vi "_CSM Message Communication Panel.vi"() -> ()   [LabVIEW 2017]
uses:
  user.lib/_NEVSTOP/Communicable State Machine(CSM)/_Support/Typedef/_CSM_GlobalLog_MSG.ctl
  user.lib/_NEVSTOP/Communicable State Machine(CSM)/_Support/Typedef/_CSM_Response Source Message.ctl
  user.lib/_NEVSTOP/Communicable State Machine(CSM)/_Support/Typedef/_CSM_GlobalLog_MSG_TYPE.ctl
  user.lib/_NEVSTOP/Communicable State Machine(CSM)/_Polymophic/Add State(s) to Queue By BOOL(Element).vi
  230fd0d1-fada-4a8e-b720-9cb1801ca748.vi
  70dded23-6362-40d9-8646-ef12445fa2f7.vi
  user.lib/_NEVSTOP/Communicable State Machine(CSM)/_Polymophic/Build Synchronous Message with Arguments.vi
  user.lib/_NEVSTOP/Communicable State Machine(CSM)/_Polymophic/Build No-Reply Asynchronous Message with Arguments.vi
  user.lib/_NEVSTOP/Communicable State Machine(CSM)/AdvanceAPI/CSM - Keywords.vi
  user.lib/_NEVSTOP/Communicable State Machine(CSM)/AdvanceAPI/CSM - Convert Error to Argument.vi
  user.lib/_NEVSTOP/Communicable State Machine(CSM)/_Support/GlobalEvent/GEvt-Generate with Rule Check.vi
  user.lib/_NEVSTOP/Communicable State Machine(CSM)/_Support/Message/Parse State with Arguments String.vi
  <vilib>/Utility/config.llb/Close Config Data.vi
  <vilib>/Utility/config.llb/Write Key.vi
  <vilib>/Utility/config.llb/Write Key (Double).vi
  <vilib>/Utility/config.llb/Write Key (I32).vi
  <vilib>/Utility/config.llb/Write Key (String).vi
  user.lib/_NEVSTOP/Communicable State Machine(CSM)/_csmHelper/lvcsmFile/Path to lvcsm String.vi
  <vilib>/Utility/config.llb/Remove Key.vi
  <vilib>/Utility/config.llb/Get Key Names.vi
  <vilib>/Utility/Data Type/Get Type Information.vi
  <vilib>/Utility/Data Type/Get Array Information.vi
  <vilib>/Utility/config.llb/Write Key (Boolean).vi
  <vilib>/Utility/config.llb/Open Config Data.vi
  user.lib/_NEVSTOP/Communicable State Machine(CSM)/_csmHelper/lvcsmFile/lvcsm File Path.vi
  user.lib/_NEVSTOP/Communicable State Machine(CSM)/_csmHelper/lvcsmFile/_Array of VData to VCluster.vi
  <vilib>/Utility/config.llb/Read Key.vi
  <vilib>/Utility/config.llb/Read Key (Double).vi
  <vilib>/Utility/config.llb/Read Key (I32).vi
  user.lib/_NEVSTOP/Communicable State Machine(CSM)/_csmHelper/lvcsmFile/lvcsm String to Path.vi
  <vilib>/Utility/config.llb/Read Key (String).vi
  <vilib>/Utility/config.llb/Read Key (Boolean).vi
  user.lib/_NEVSTOP/Communicable State Machine(CSM)/_Support/GlobalEvent/LogFilter/LogFilter - Check.vi
  user.lib/_NEVSTOP/Communicable State Machine(CSM)/_Support/GlobalEvent/Cache-GEvt Refs.vi
  user.lib/_NEVSTOP/Communicable State Machine(CSM)/_Support/GlobalEvent/LogFilter/LogFilter.lvclass
  user.lib/_NEVSTOP/Communicable State Machine(CSM)/Communicable State Machine.lvlib
  user.lib/_NEVSTOP/Communicable State Machine(CSM)/_Shared/CSM Shared.lvlib
panel:
  in  "History":i32(listbox)
  in  "CSM 2":string(combo)
  in  "Refresh":bool
  in  "Arguments":string
  out "Response":string
  in  "Clear History":bool
  in  "History Length":i32=50 min=20 max=1000 step=1
  in  "CSM":string(combo)
  in  "Refresh CSM":bool
  in  "RespTMO(ms)":i32=10000 format="%.0p"
  in  "Sync (-@) 2":bool
  in  "Sync (-@)":bool
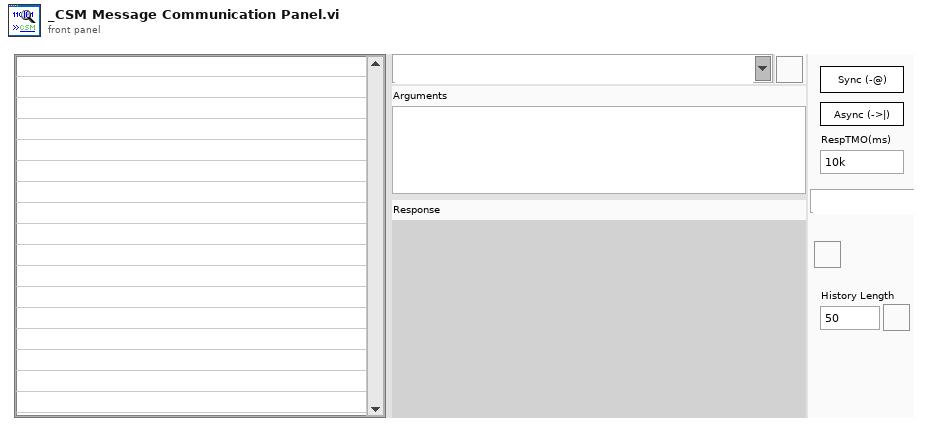
[diagram p1: front panel]
types:
  T1 = enum32{"Invalid", "Standard", "Closed", "Hidden", "Minimized", "Maximized"}
  T2 = enum32{"invalid app kind", "Development System", "Run Time System", "Student Edition", "Embedded LabVIEW", "Evaluation", "Custom"}
  T3 = cluster{"Response Timeout(ms)":i32, "History Length":i32, "History":string[]}
  T4 = cluster{"Shift":bool, "Ctrl":bool, "Alt":bool, "Cmd":bool, "Opt":bool}
  T5 = cluster{"Core":cluster{"Current VI Reference":refnum<vi>, "Close Panel on Exit?":bool}, "CSM Global Log Event":refnum<user-event>, "MessageList":string[], "Toobar.advance":refnum<vi>[]}
  T6 = typedef "LVPoint32TypeDef.ctl" = cluster{"Horizontal":i32, "Vertical":i32}
  T7 = cluster{"Current VI Reference":refnum<vi>, "Close Panel on Exit?":bool}
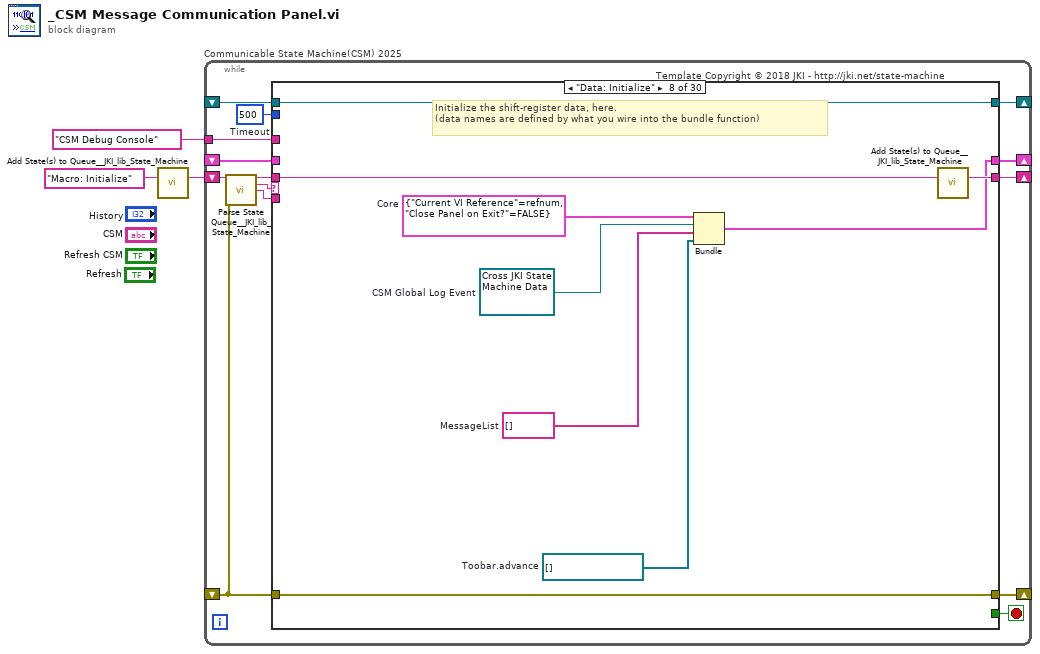
[diagram p0: block diagram]
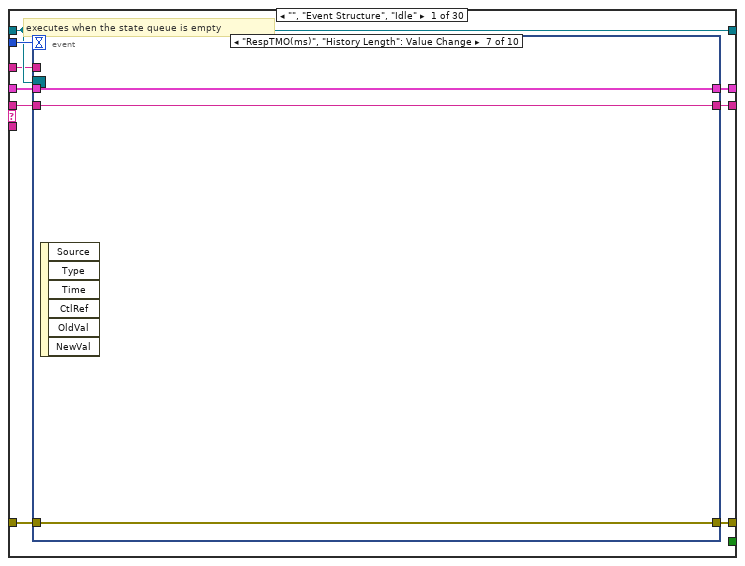
[diagram p2: hidden frame]
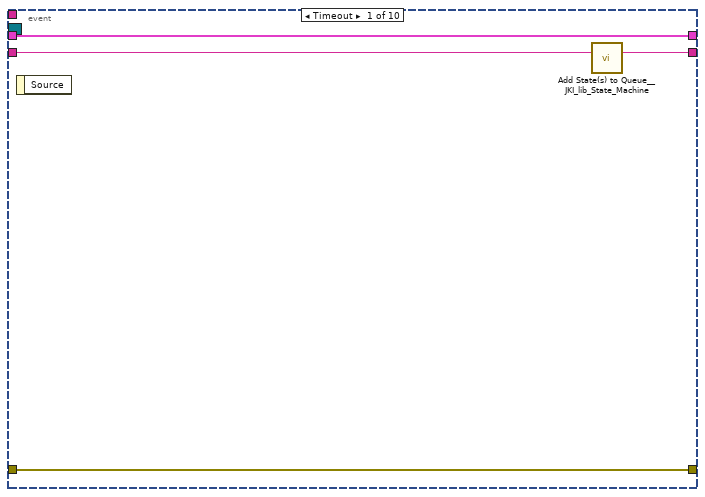
[diagram p3: hidden frame]
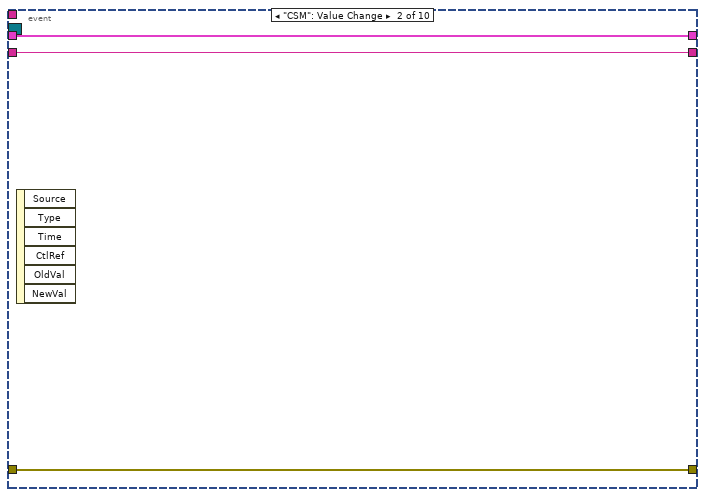
[diagram p4: hidden frame]
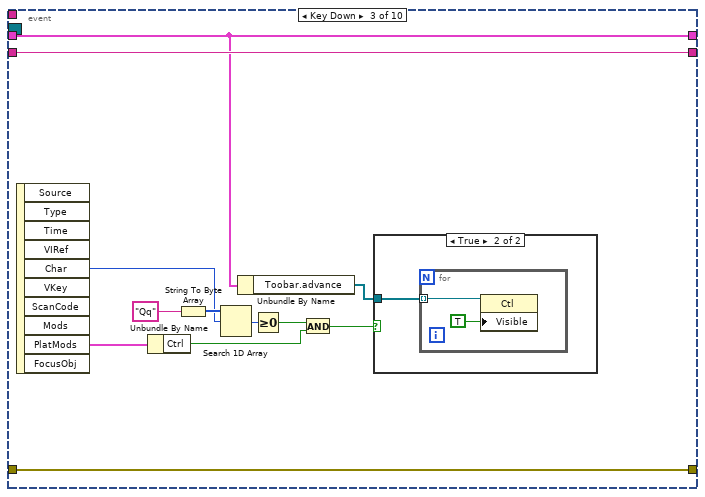
[diagram p5: hidden frame]
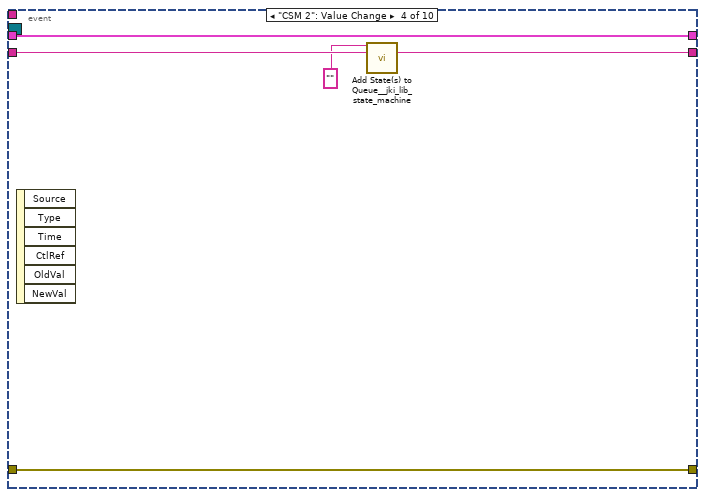
[diagram p7: hidden frame]
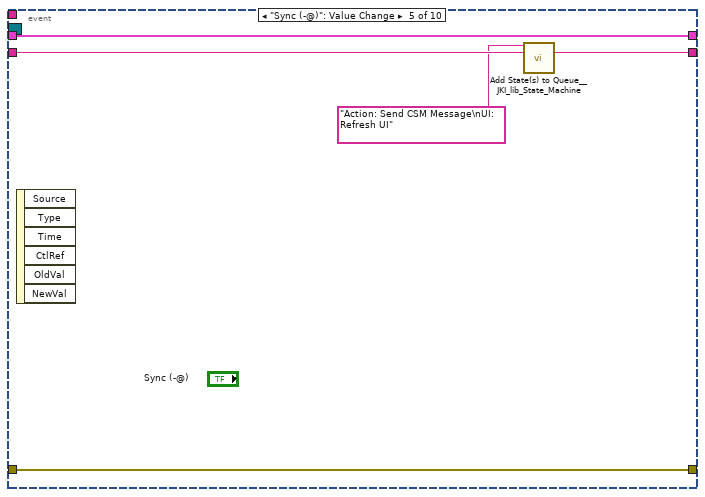
[diagram p8: hidden frame]
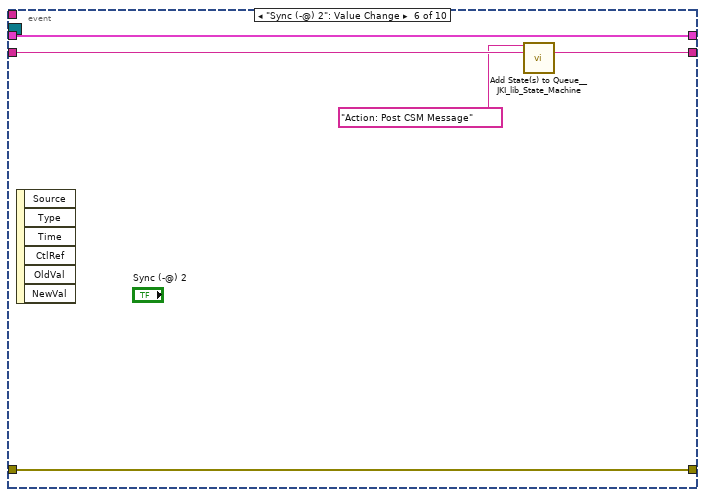
[diagram p9: hidden frame]
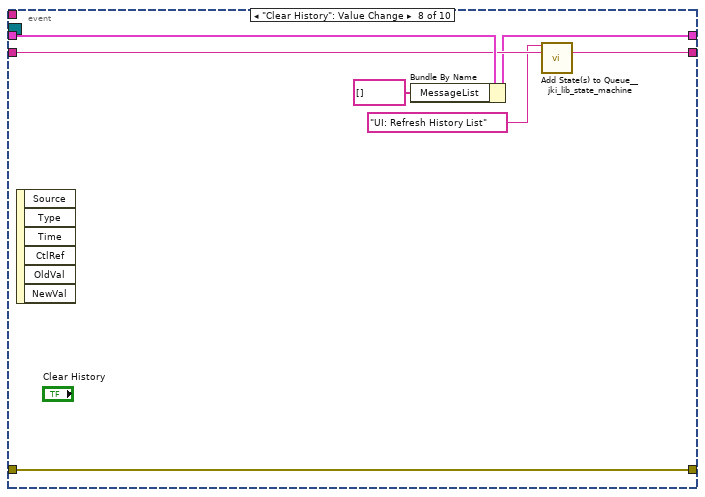
[diagram p10: hidden frame]
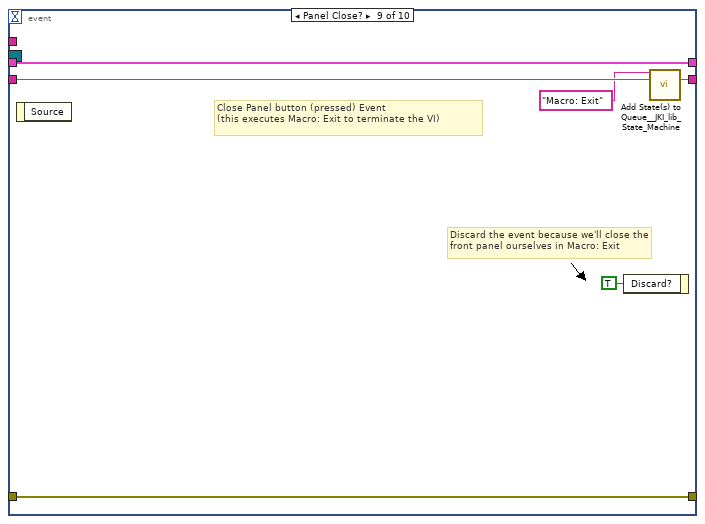
[diagram p11: hidden frame]
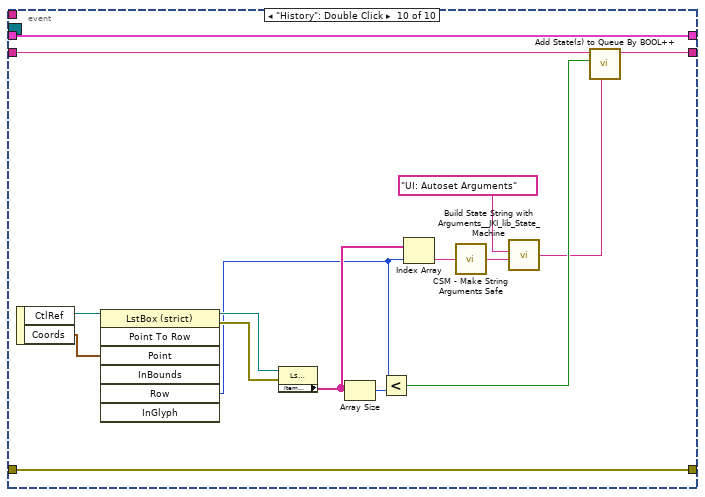
[diagram p12: hidden frame]
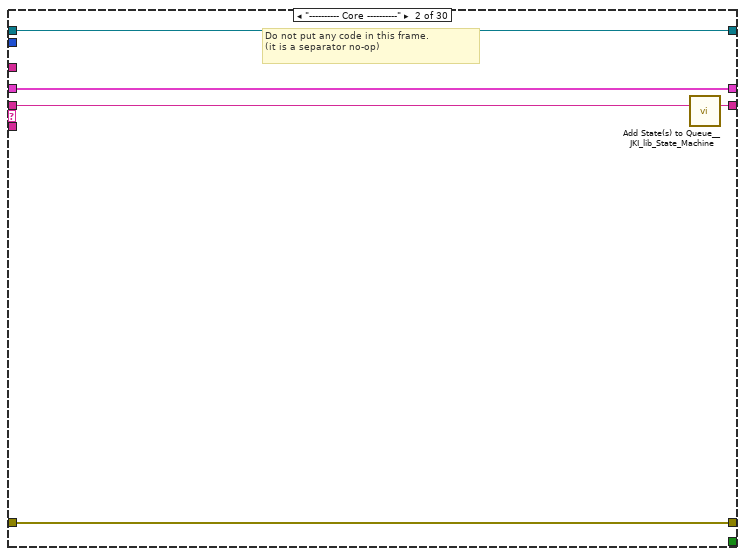
[diagram p13: hidden frame]
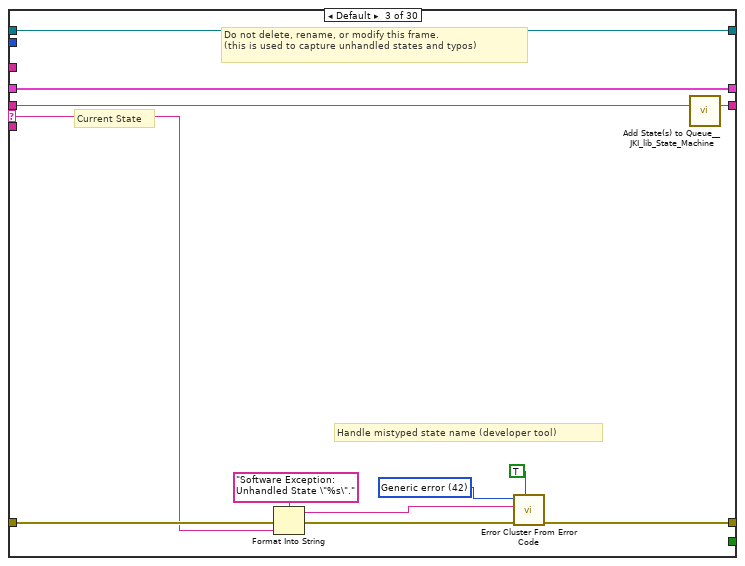
[diagram p14: hidden frame]
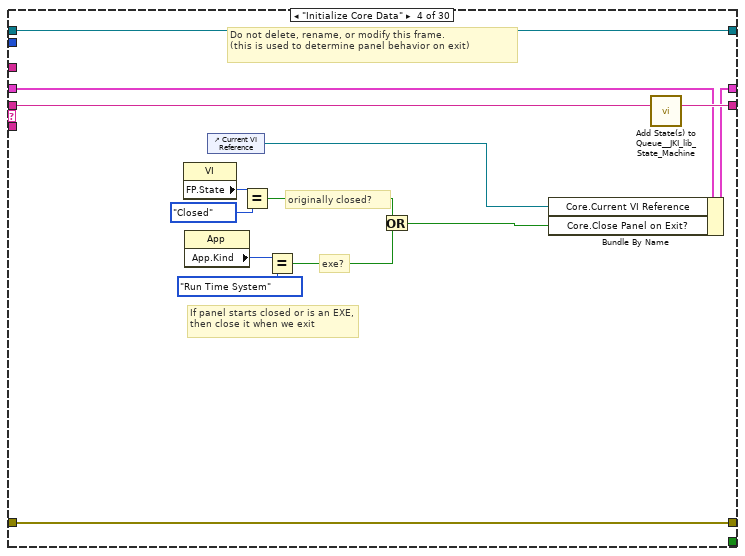
[diagram p15: hidden frame]
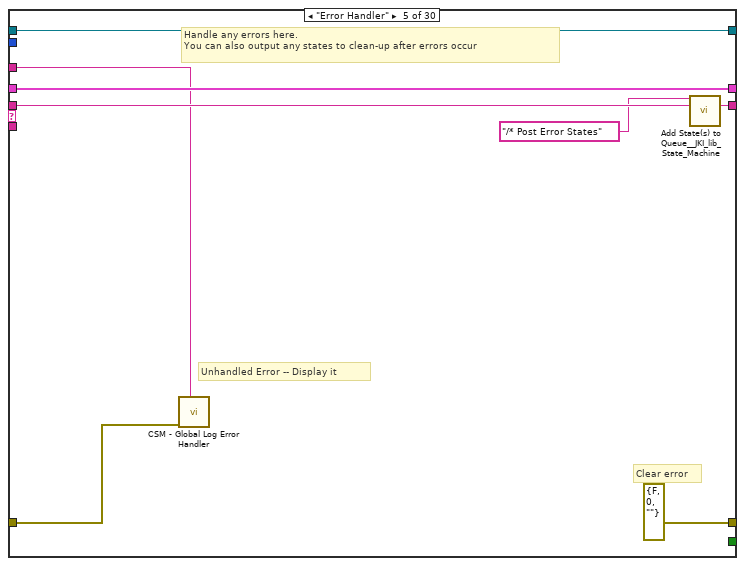
[diagram p16: hidden frame]
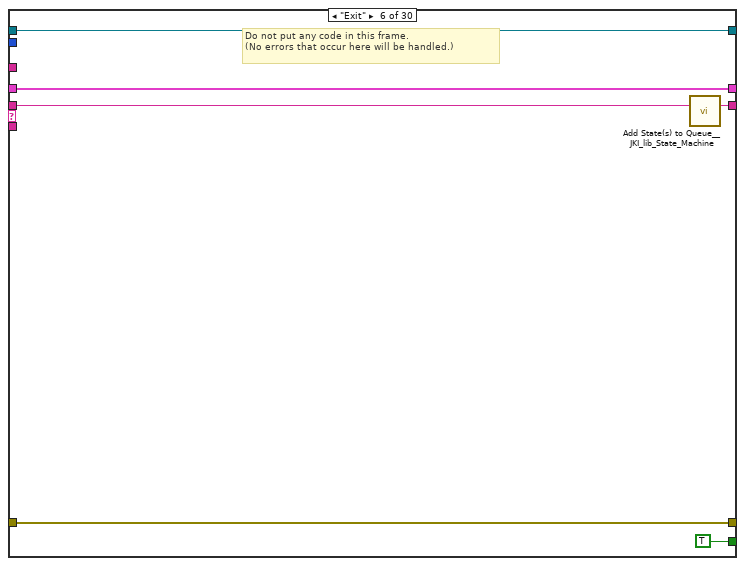
[diagram p17: hidden frame]
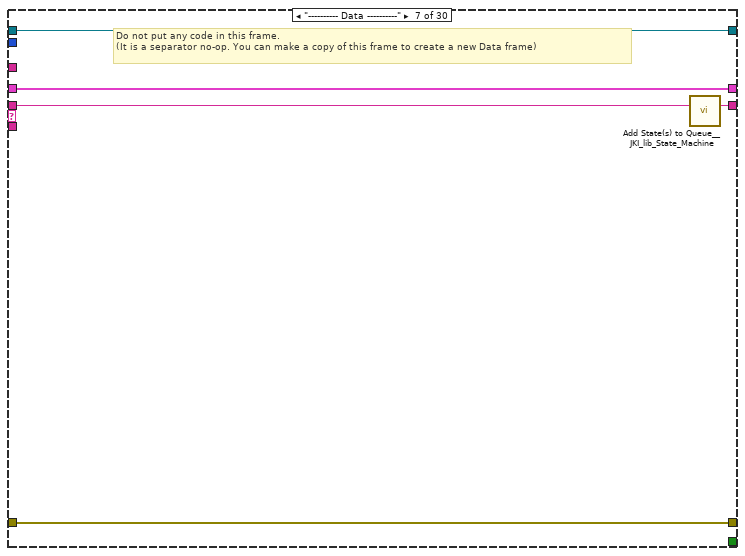
[diagram p18: hidden frame]
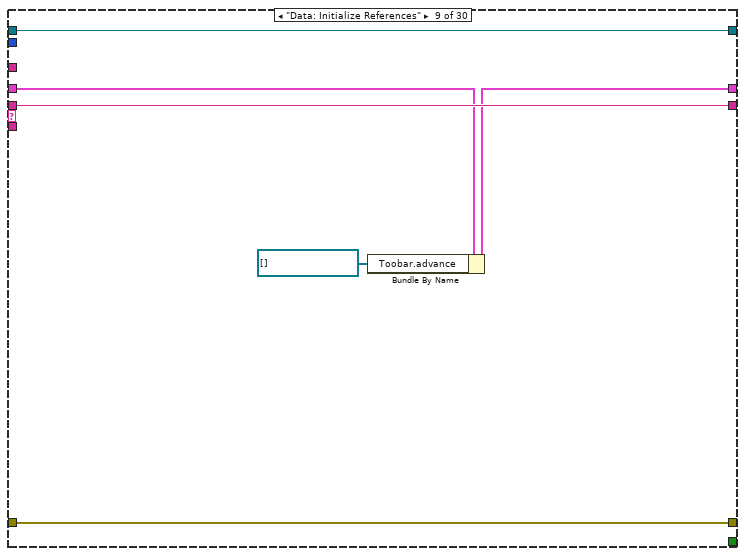
[diagram p19: hidden frame]
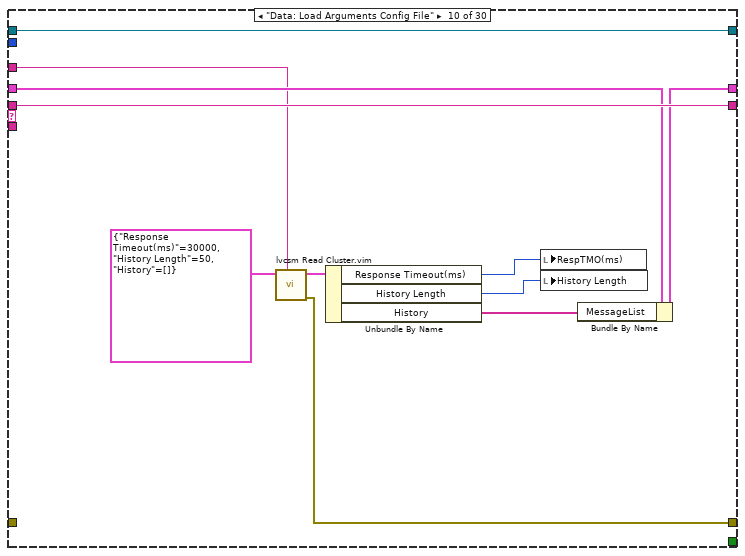
[diagram p20: hidden frame]
diagram:
  n1 = call <vilib>:"Add State(s) to Queue__JKI_lib_State_Machine.vi"("State(s) in (\"\")"="Macro: Initialize") -> ("States Out"=w2:string)  [unwired: 14 in]
  n2 = while "Communicable State Machine(CSM) 2025" {
    shift-right: [w10] -> _
    shift-left: _ -> [w9]
    shift-right: [w13] -> _
    shift-left: _ -> [w7]
    shift-right: [w12] -> _
    shift-left: w2 -> [w14]
    shift-right: [w6] -> _
    shift-left: _ -> [w5]
    tunnel: "CSM Debug Console" -> [w4]
    stop <- w11 stop-if-true
    w8 = 500  # Timeout
    # "Template Copyright © 2018 JKI - http://jki.net/state-machine"
    n3 = call <vilib>:"Parse State Queue__JKI_lib_State_Machine.vi"("State Queue"=w14, "Error In (no error)"=w7) -> ("Remaining States"=w16:string, "Current State"=w17:string, "Arguments"=w15:string)  [unwired: 11 in]
    n4 = case shown="\"Data: Initialize\"" w17 {
      selector: w17 -> [_ _ w102 _ _ _ _ _ _ _ _ _ _ _ _ _ _ _ _ _ _ _ _ _ _ _ _ _ _ _]
      tunnel: w16 -> [w26 w100 w106 w126 w134 w140 w145 w154 w159 w171 w181 w194 w210 w215 w222 w229 w234 w240 w250 w262 w341 w352 w365 w369 w375 w381 w392 w397 w407 w429]
      tunnel: w15 -> [_ _ _ _ _ _ _ _ _ _ _ w189 _ _ _ _ _ _ w245 w256 w339 _ _ _ _ _ _ _ _ _]
      tunnel: w9 -> [w24 w97 w104 w119 w131 w138 w142 _ w158 w168 w179 w191 w205 w212 w220 w225 w231 w236 w248 w258 w336 w350 w364 w367 w372 w378 w389 w394 w405 w427]
      tunnel: [w23 w98 w108 w123 errorcluster {"status"=FALSE, "code"=0, "source"=""} ("error out") w137 w143 w151 w160 w164 w174 w192 w206 w213 w218 w226 w232 w238 w246 w259 w342 w353 w366 w370 w373 w379 w390 w395 w401 w425] -> w13
      tunnel: w7 -> [w22 w98 w107 w123 w130 w137 w143 w151 w160 _ _ w192 w207 w213 _ _ w232 w238 w247 w260 w342 w353 w366 w370 w373 w379 w390 w395 _ _]
      tunnel: [w25 w99 w105 w125 w133 w139 w144 w153 w159 w171 w181 w194 w209 w214 w221 w228 w233 w239 w249 w261 w341 w352 w365 w369 w374 w380 w391 w396 w406 w428] -> w12
      tunnel: [_ _ _ _ _ TRUE _ _ _ _ _ _ _ _ _ _ _ _ _ _ _ _ _ _ _ _ _ _ _ _] -> w11
      tunnel: [w21 w97 w104 w124 w131 w138 w142 w152 w156 w169 w179 w185 w205 w212 w220 w225 w231 w236 w248 w258 w336 w350 w364 w367 w372 w378 w389 w394 w405 w427] -> w10
      tunnel: w8 -> [w20 _ _ _ _ _ _ _ _ _ _ _ _ _ _ _ _ _ _ _ _ _ _ _ _ _ _ _ _ _]
      tunnel: [w19 w96 w101 w113 w128 w135 w141 w149 w157 w170 w180 w193 w204 w211 w219 w227 w230 w237 w244 w255 w340 w351 w363 w368 w371 w376 w382 w393 w404 w426] -> w6
      tunnel: w5 -> [w19 w96 w101 w113 w128 w135 w141 w149 w157 w170 w180 w193 w204 w211 _ w227 w230 w237 w244 w255 w340 w351 w363 w368 w371 w376 w382 w393 w404 w426]
      tunnel: w4 -> [w18 _ _ _ w127 _ _ _ _ w163 w175 _ _ _ _ _ _ _ _ _ _ _ _ _ _ _ _ _ _ _]
      frame "", "Event Structure", "Idle" {
        # "executes when the state queue is empty"
        n5 = event shown="[6] \"RespTMO(ms)\", \"History Length\": Value Change" {
          selector: w19 -> [_ _ _ _ _ _ _ _ _ _]
          dyn-events: _ -> [_ _ _ _ _ _ _ _ _ _]
          timeout: w20 -> [_ _ _ _ _ _ _ _ _ _]
          tunnel: w26 -> [w30 w33 w45 w50 w55 w60 w66 w70 w79 w87]
          tunnel: [w29 w33 w45 w51 w56 w61 w66 w71 w78 w88] -> w25
          tunnel: w24 -> [w27 w31 w34 w52 w57 w62 w64 w72 w76 w94]
          tunnel: [w28 w32 w44 w53 w58 w63 w65 w73 w77 w95] -> w23
          tunnel: w22 -> [w28 w32 w44 w53 w58 w63 w65 w73 w77 w95]
          tunnel: [w27 w31 w34 w52 w57 w62 w64 w68 w76 w94] -> w21
          tunnel: w18 -> [_ _ _ _ _ _ _ _ _ _]
          event Timeout {
            n6 = event-data() -> ()  [unwired: 1 in, 1 out]
            n7 = call <vilib>:"Add State(s) to Queue__JKI_lib_State_Machine.vi"("State(s) in (\"\")"=w30) -> ("States Out"=w29:string)  [unwired: 14 in]
          }
          event "CSM": Value Change {
            n8 = event-data() -> ()  [unwired: 1 in, 6 out]
          }
          event Key Down {
            n9 = event-data() -> ("Char"=w35:i16, "PlatMods"=w36:T4)  [unwired: 1 in, 8 out]
            n10 = Unbundle By Name(w36) -> ("Ctrl"=w39:bool)
            n11 = String To Byte Array(string="Qq") -> (unsigned byte array=w41:u8[])
            n12 = Search 1D Array(1D array=w41, element=w35) -> (index of element=w42:i32)  [unwired: 1 in]
            n13 = Unbundle By Name(w34) -> ("Toobar.advance"=w37:refnum<vi>[])
            n14 = Greater Or Equal To 0?(x=w42) -> (x >= 0?=w43:bool)
            n15 = And(x=w43, y=w39) -> (x .and. y?=w38:bool)
            n16 = case shown="True" w38 {
              tunnel: w37 -> [_ w46]
              frame False {
              }
              frame True {
                n17 = for {
                  tunnel: w46 -> [w48] mode=indexing
                  n18 = property class="Ctl"(reference=w48, "Visible"=TRUE) -> ()  [unwired: 1 in, 2 out]
                }
              }
            }
          }
          event "CSM 2": Value Change {
            n19 = event-data() -> ()  [unwired: 1 in, 6 out]
            n20 = call <vilib>:"Add State(s) to Queue__jki_lib_state_machine.vi"("State(s) in Front (\"\")"="" ("State(s) in Front (\"\")"), "State(s) in (\"\")"=w50) -> ("States Out"=w51:string)  [unwired: 13 in]
          }
          event "Sync (-@)": Value Change {
            n21 = event-data() -> ()  [unwired: 1 in, 6 out]
            n22 = call <vilib>:"Add State(s) to Queue__JKI_lib_State_Machine.vi"("State(s) in Front (\"\")"="Action: Send CSM Message\nUI: Refresh UI" ("State(s) in Front (\"\")"), "State(s) in (\"\")"=w55) -> ("States Out"=w56:string)  [unwired: 13 in]
          }
          event "Sync (-@) 2": Value Change {
            n23 = event-data() -> ()  [unwired: 1 in, 6 out]
            n24 = call <vilib>:"Add State(s) to Queue__JKI_lib_State_Machine.vi"("State(s) in Front (\"\")"="Action: Post CSM Message" ("State(s) in Front (\"\")"), "State(s) in (\"\")"=w60) -> ("States Out"=w61:string)  [unwired: 13 in]
          }
          event "RespTMO(ms)", "History Length": Value Change {
            n25 = event-data() -> ()  [unwired: 1 in, 6 out]
          }
          event "Clear History": Value Change {
            n26 = event-data() -> ()  [unwired: 1 in, 6 out]
            n27 = Bundle By Name(cluster=w72, "MessageList"=string[] []) -> (w68:T5)
            n28 = call <vilib>:"Add State(s) to Queue__jki_lib_state_machine.vi"("State(s) in Front (\"\")"="UI: Refresh History List" ("State(s) in Front (\"\")"), "State(s) in (\"\")"=w70) -> ("States Out"=w71:string)  [unwired: 13 in]
          }
          event Panel Close? {
            # "Discard the event because we'll close the front panel ourselves in Macro: Exit"
            # "Close Panel button (pressed) Event\n(this executes Macro: Exit to terminate the VI)"
            n29 = event-data() -> ()  [unwired: 1 in, 1 out]
            n30 = event-data("Discard?"=TRUE) -> ()  [unwired: 1 in, 1 out]
            n31 = call <vilib>:"Add State(s) to Queue__JKI_lib_State_Machine.vi"("State(s) in Front (\"\")"="Macro: Exit", "State(s) in (\"\")"=w79) -> ("States Out"=w78:string)  [unwired: 13 in]
          }
          event "History": Double Click {
            n32 = event-data() -> ("CtlRef"=w93:refnum<vi>, "Coords"=w81:T6)  [unwired: 1 in]
            n33 = invoke class="LstBox (strict)" method="Point To Row"(reference=w93, "Point"=w81) -> (reference out=w92:refnum<vi>, error out=w91:errorcluster, "Row"=w80:i32)  [unwired: 5 in, 4 out]
            n34 = property class="LstBox (strict)"(reference=w92, error in=w91) -> ("Item Names"=w89:string[])  [unwired: 2 out]
            n35 = Array Size(array=w89) -> (size(s)=w90:i32)
            n36 = Less?(x=w80, y=w90) -> (x < y?=w86:bool)
            n37 = Index Array(array=w89, index=w80) -> (element=w85:string)
            n38 = call "CSM - Make String Arguments Safe.vi"("Argurment String"=w85) -> ("Safe Argurment String"=w84:string)  [unwired: 8 in]
            n39 = call <vilib>:"Build State String with Arguments__JKI_lib_State_Machine.vi"("Arguments (\"\")"=w84, "State"="UI: Autoset Arguments") -> ("State with Arguments"=w82:string)  [unwired: 4 in]
            n40 = call-poly "Add State(s) to Queue By BOOL++.vi"("TRUE (\"\")"=w82, "Condition"=w86, "State Queue (\"\")"=w87) -> ("Remaining States"=w88:string)  [unwired: 8 in]
          }
        }
      }
      frame "---------- Core ----------" {
        # "Do not put any code in this frame.\n(it is a separator no-op)"
        n41 = call <vilib>:"Add State(s) to Queue__JKI_lib_State_Machine.vi"("State(s) in (\"\")"=w100) -> ("States Out"=w99:string)  [unwired: 14 in]
      }
      frame Default {
        w111 = 42 items=["No error", "Argument error", "Memory is full", "Out of zone", "End of file", "File already open", "Generic file I/O error", "File not found", "File permission error", "Disk is full", "Duplicate path", "Too many files open", "System feature not enabled", "Resource file not found", "Cannot add resource", "Resource not found", "Image not found", "Image memory error", "Pen does not exist", "Config type invalid", "Config token not found", "Config parse error", "Config memory error", "Bad external code format", "Bad external code offset", "External code not present", "Null window", "Destroy window error", "Null menu", "Print aborted", "Bad print record", "Print driver error", "Windows error during printing", "Memory error during printing", "Print dialog error", "Generic print error", "Invalid device refnum", "Device not found", "Device parameter error", "Device unit error", "Cannot open device", "Device call aborted", "Generic error", "Cancelled by user", "Object ID too low", "Object ID too high", "Object not in heap", "Unknown heap", "Unknown object (invalid DefProc)", "Unknown object (DefProc not in table)", "Message out of range", "Invalid (null) method", "Unknown message", "Manager call not supported", "Bad address", "Network operation in progress", "Network operation timed out", "Connection is busy", "Network attribute not supported", "Network error", "Address in use", "System out of memory", "Connection aborted", "Connection refused", "Not connected", "Already connected", "Connection closed", "Initialization error (interapplication manager)", "Bad occurrence", "Wait on unbound occurrence handler", "Occurrence queue overflow", "Datalog type conflict", "Unused", "Unrecognized type (interapplication manager)", "Memory corrupt", "Failed to make temporary DLL", "Old CIN version", "Drag socket not found", "Failed to load drop-object", "Failed to register OLE object", "Failed to release OLE object", "Format specifier type mismatch", "Unknown format specifier", "Too few format specifiers", "Too many format specifiers", "Scan failed", "Newer CIN version", "Error converting to variant", "Runtime menu error", "Password tampered", "Variant attribute not found", "Incompatible variant data type", "Event data is not available", "Event Store is not present", "Occurrence is not found", "Event Queue is not created", "Event info is not available", "Refnum passed is NULL", "Error retrieving Class GUID", "Error retrieving CoClass GUID", "Error retrieving TypeLib GUID.", "Bad built application magic bytes.", "Specific driver is different from the specific driver associated with the Logical Name.", "There is no session opened to the class driver.", "Max Error", "MAX - Error with config objects", "MAX - Error loading configuration", "MAX - Group not supported"]
        # "Current State"
        # "Do not delete, rename, or modify this frame.\n(this is used to capture unhandled states and typos)"
        # "Handle mistyped state name (developer tool)"
        n42 = Format Into String(format string="Software Exception: Unhandled State \"%s\"." ("message"), error in=w107, w102) -> (resulting string=w110:string, error out=w109:errorcluster)  [unwired: 1 in]
        n43 = call <vilib>:"Error Cluster From Error Code.vi"("show call chain? (False)"=TRUE, "error in (no error)"=w109, "error message (\"\")"=w110, "error code (0)"=w111) -> ("error out"=w108:errorcluster)  [unwired: 5 in]
        n44 = call <vilib>:"Add State(s) to Queue__JKI_lib_State_Machine.vi"("State(s) in (\"\")"=w106) -> ("States Out"=w105:string)  [unwired: 14 in]
      }
      frame "Initialize Core Data" {
        # "Do not delete, rename, or modify this frame.\n(this is used to determine panel behavior on exit)"
        # "originally closed?"
        # "exe?"
        # "If panel starts closed or is an EXE, then close it when we exit"
        n45 = property class="VI"() -> ("FP.State"=w116:T1)  [unwired: 2 in, 2 out]
        n46 = property class="App"() -> ("App.Kind"=w122:T2)  [unwired: 2 in, 2 out]
        n47 = control-ref of="Current VI Reference"() -> (w117:refnum<vi>)
        n48 = Equal?(x=w116, y=T1."Closed" ("Front Panel Window:State")) -> (x = y?=w114:bool)
        n49 = Equal?(x=w122, y=T2."Run Time System" ("Application:Kind")) -> (x = y?=w120:bool)
        n50 = Or(x=w114, y=w120) -> (x .or. y?=w118:bool)
        n51 = Bundle By Name(cluster=w119, "Core.Current VI Reference"=w117, "Core.Close Panel on Exit?"=w118) -> (w124:T5)
        n52 = call <vilib>:"Add State(s) to Queue__JKI_lib_State_Machine.vi"("State(s) in (\"\")"=w126) -> ("States Out"=w125:string)  [unwired: 14 in]
      }
      frame "Error Handler" {
        # "Unhandled Error -- Display it"
        # "Handle any errors here.\nYou can also output any states to clean-up after errors occur"
        # "Clear error"
        n53 = call "CSM - Global Log Error Handler.vi"("Place (\"\" to Use VI's Name)"=w127, "Error In"=w130) -> ()  [unwired: 9 in, 1 out]
        n54 = call <vilib>:"Add State(s) to Queue__JKI_lib_State_Machine.vi"("State(s) in Front (\"\")"="/* Post Error States", "State(s) in (\"\")"=w134) -> ("States Out"=w133:string)  [unwired: 13 in]
      }
      frame "Exit" {
        # "Do not put any code in this frame.\n(No errors that occur here will be handled.)"
        n55 = call <vilib>:"Add State(s) to Queue__JKI_lib_State_Machine.vi"("State(s) in (\"\")"=w140) -> ("States Out"=w139:string)  [unwired: 14 in]
      }
      frame "---------- Data ----------" {
        # "Do not put any code in this frame.\n(It is a separator no-op. You can make a copy of this frame to create a new Data frame)"
        n56 = call <vilib>:"Add State(s) to Queue__JKI_lib_State_Machine.vi"("State(s) in (\"\")"=w145) -> ("States Out"=w144:string)  [unwired: 14 in]
      }
      frame "Data: Initialize" {
        w146 = refnum<vi>[] []  # Toobar.advance
        w147 = string[] []  # MessageList
        w148 = refnum<user-event> refnum  # CSM Global Log Event
        w150 = T7 {"Current VI Reference"=refnum, "Close Panel on Exit?"=FALSE}  # Core
        # "Initialize the shift-register data, here.\n(data names are defined by what you wire into the bundle function)"
        n57 = Bundle("Core"=w150, "CSM Global Log Event"=w148, "MessageList"=w147, "Toobar.advance"=w146) -> (w152:T5)  [unwired: 1 in]
        n58 = call <vilib>:"Add State(s) to Queue__JKI_lib_State_Machine.vi"("State(s) in (\"\")"=w154) -> ("States Out"=w153:string)  [unwired: 14 in]
      }
      frame "Data: Initialize References" {
        n59 = Bundle By Name(cluster=w158, "Toobar.advance"=refnum<vi>[] []) -> (w156:T5)
      }
      frame "Data: Load Arguments Config File" {
        n60 = call "lvcsm Read Cluster.vim"("Section"=w163, "Default Prototype"=T3 {"Response Timeout(ms)"=30000, "History Length"=50, "History"=[]}) -> ("error out"=w164:errorcluster, "Cluster (Dup)"=w167:T3)  [unwired: 8 in]
        n61 = Unbundle By Name(w167) -> ("Response Timeout(ms)"=w162:i32, "History Length"=w161:i32, "History"=w165:string[])
        n62 = local write "RespTMO(ms)"(w162) -> ()
        n63 = local write "History Length"(w161) -> ()
        n64 = Bundle By Name(cluster=w168, "MessageList"=w165) -> (w169:T5)
      }
      frame "Data: Save Arguments Config File" {
        n65 = Unbundle By Name(w179) -> ("MessageList"=w176:string[])
        n66 = local read "RespTMO(ms)"() -> (w173:i32)
        n67 = local read "History Length"() -> (w172:i32)
        n68 = Bundle By Name(cluster=T3 {"Response Timeout(ms)"=30000, "History Length"=50, "History"=[]}, "History"=w176, "Response Timeout(ms)"=w173, "History Length"=w172) -> (w178:T3)
        n69 = call "lvcsm Write Cluster.vim"("Section"=w175, "Configuration"=w178) -> ("error out"=w174:errorcluster)  [unwired: 9 in]
      }
      frame "Data: Update Message List" {
        n70 = Unbundle By Name(w191) -> ("MessageList"=w190:string[])
        n71 = call "CSM - Revert Arguments-Safe String.vi"("Safe Argurment String"=w189) -> ("Origin Argurment String"=w188:string)  [unwired: 8 in]
        n72 = Build Array (concatenate)(w188, w190) -> (w187:string[])
        n73 = for {
          tunnel: w187 -> [w198] mode=indexing
          shift-right: [w197] -> w183
          shift-left: string[] [] -> [w196]
          i -> [w195]
          n74 = Search 1D Array(1D array=w196, element=w198) -> (index of element=w199:i32)  [unwired: 1 in]
          n75 = case shown="-1" w199 {
            tunnel: w198 -> [_ w203]
            tunnel: [w200 w201] -> w197
            tunnel: w196 -> [w200 w202]
            tunnel: w195 -> [_ _]
            frame Default {
            }
            frame -1 {
              n76 = Build Array (concatenate)(w202, w203) -> (w201:string[])
            }
          }
        }
        n77 = Array Subset(array=w183, length="History Length") -> (w184:string[])  [unwired: 1 in]
        n78 = Bundle By Name(cluster=w191, "MessageList"=w184) -> (w185:T5)
      }
      frame "Data: Cleanup" {
        # "Cleanup any data and references, here.\n(this is called automatically, by the Macro: Exit)"
        n79 = Unbundle By Name(w205) -> ("Core.Current VI Reference"=w208:refnum<vi>)
        n80 = Close Reference(reference=w208, error in (no error)=w207) -> (error out=w206:errorcluster)
        n81 = call <vilib>:"Add State(s) to Queue__JKI_lib_State_Machine.vi"("State(s) in (\"\")"=w210) -> ("States Out"=w209:string)  [unwired: 14 in]
      }
      frame "---------- Events ----------" {
        # "Do not put any code in this frame.\n(It is a separator no-op. You can make a copy of this frame to create a new UI frame)"
        n82 = call <vilib>:"Add State(s) to Queue__JKI_lib_State_Machine.vi"("State(s) in (\"\")"=w215) -> ("States Out"=w214:string)  [unwired: 14 in]
      }
      frame "Events: Register" {
        # "Do not put any code in this frame.\n(It is a separator no-op. You can make a copy of this frame to create a new UI frame)"
        n83 = call "CSM - Global Log Event.vi"() -> ("error out"=w216:errorcluster, "CSM Global Log Event"=w217:refnum<user-event>)  [unwired: 10 in]
        n84 = register-events(error in=w216, w217) -> (reference out=w219:refnum<event-registration>, error out=w218:errorcluster)  [unwired: 1 in]
        n85 = call <vilib>:"Add State(s) to Queue__JKI_lib_State_Machine.vi"("State(s) in (\"\")"=w222) -> ("States Out"=w221:string)  [unwired: 14 in]
      }
      frame "Events: Unregister" {
        # "Do not put any code in this frame.\n(It is a separator no-op. You can make a copy of this frame to create a new UI frame)"
        n86 = Unbundle By Name(w225) -> ("CSM Global Log Event"=w224:refnum<user-event>)
        n87 = call "CSM - Destroy Global Log Event.vi"("CSM Global Log Event"=w224) -> ("error out"=w223:errorcluster)  [unwired: 10 in]
        n88 = Unregister For Events(event registration refnum=w227, error in=w223) -> (error out=w226:errorcluster)
        n89 = call <vilib>:"Add State(s) to Queue__JKI_lib_State_Machine.vi"("State(s) in (\"\")"=w229) -> ("States Out"=w228:string)  [unwired: 14 in]
      }
      frame "---------- UI ----------" {
        # "Do not put any code in this frame.\n(It is a separator no-op. You can make a copy of this frame to create a new UI frame)"
        n90 = call <vilib>:"Add State(s) to Queue__JKI_lib_State_Machine.vi"("State(s) in (\"\")"=w234) -> ("States Out"=w233:string)  [unwired: 14 in]
      }
      frame "UI: Initialize" {
        # "Initialize the User Interface, here.\n(this is called automatically, by the Macro: Init)"
        n91 = Unbundle By Name(w236) -> ("Toobar.advance"=w235:refnum<vi>[])
        n92 = disable-structure shown="Disabled" {
          disable-tunnel: w235 -> [w241 _]
          frame Disabled {
            n93 = for {
              tunnel: w241 -> [w243] mode=indexing
              n94 = property class="Ctl"(reference=w243, "Visible"=FALSE) -> ()  [unwired: 1 in, 2 out]
            }
          }
          frame Enabled {
          }
        }
        n95 = call <vilib>:"Add State(s) to Queue__JKI_lib_State_Machine.vi"("State(s) in (\"\")"=w240) -> ("States Out"=w239:string)  [unwired: 14 in]
      }
      frame "UI: Cursor Set" {
        # "Argument"
        # "Set and Unset Cursor Busy.\n(Usage: \"UI: Cursor Set >> Busy|Idle\")"
        n96 = case shown="\"Idle\", Default" w245 {
          tunnel: w247 -> [w252 w254]
          tunnel: [w251 w253] -> w246
          frame "Idle", Default {
            n97 = call <vilib>:"Unset Busy.vi"("error in (no error)"=w252) -> ("error out"=w251:errorcluster)  [unwired: 10 in]
          }
          frame "Busy" {
            n98 = call <vilib>:"Set Busy.vi"("error in (no error)"=w254) -> ("error out"=w253:errorcluster)  [unwired: 9 in, 1 out]
          }
        }
        n99 = call <vilib>:"Add State(s) to Queue__JKI_lib_State_Machine.vi"("State(s) in (\"\")"=w250) -> ("States Out"=w249:string)  [unwired: 14 in]
      }
      frame "UI: Front Panel State" {
        # "Argument"
        # "Set Front Panel Open or Closed\n(Usage: \"UI: Front Panel State >> Open|Close\")"
        n100 = Unbundle By Name(w258) -> ("Core.Current VI Reference"=w257:refnum<vi>)
        n101 = case shown="\"Minimize\", \"Minimized\"" w256 {
          tunnel: w260 -> [w268 w283 w294 w307 w320]
          tunnel: [w270 w284 w296 w309 w322] -> w259
          tunnel: w257 -> [w269 w281 w295 w308 w321]
          frame "Open", "Standard", Default {
            w263 = T1."Standard" ("State")
            n102 = property class="VI"(reference=w269, error in=w268) -> (reference out=w266:refnum<vi>, error out=w267:errorcluster, "FP.State"=w265:T1)
            n103 = Not Equal?(x=w265, y=w263) -> (x != y?=w264:bool)
            n104 = case shown="True" w264 {
              tunnel: [w274 w276] -> w270
              tunnel: w267 -> [w273 w276]
              tunnel: w266 -> [w272 _]
              tunnel: w263 -> [w271 _]
              frame True {
                n105 = invoke class="VI" method="FP.Open"(reference=w272, error in=w273, "Activate"=TRUE, "State"=w271) -> (error out=w274:errorcluster)  [unwired: 1 in, 4 out]
              }
              frame False {
              }
            }
          }
          frame "Close", "Closed" {
            n106 = property class="VI"(reference=w281, error in=w283) -> (reference out=w280:refnum<vi>, error out=w282:errorcluster, "FP.State"=w278:T1)
            n107 = Not Equal?(x=w278, y=T1."Closed" ("Front Panel Window:State")) -> (x != y?=w277:bool)
            n108 = case shown="True" w277 {
              tunnel: [w285 w288] -> w284
              tunnel: w282 -> [w285 w287]
              tunnel: w280 -> [_ w286]
              frame False {
              }
              frame True {
                n109 = invoke class="VI" method="FP.Close"(reference=w286, error in=w287) -> (error out=w288:errorcluster)  [unwired: 1 in, 2 out]
              }
            }
          }
          frame "Hidden", "Hide" {
            w289 = T1."Hidden" ("State")
            n110 = property class="VI"(reference=w295, error in=w294) -> (reference out=w292:refnum<vi>, error out=w293:errorcluster, "FP.State"=w291:T1)
            n111 = Not Equal?(x=w291, y=w289) -> (x != y?=w290:bool)
            n112 = case shown="True" w290 {
              tunnel: [w300 w301] -> w296
              tunnel: w293 -> [w299 w301]
              tunnel: w292 -> [w298 _]
              tunnel: w289 -> [w297 _]
              frame True {
                n113 = invoke class="VI" method="FP.Open"(reference=w298, error in=w299, "State"=w297) -> (error out=w300:errorcluster)  [unwired: 2 in, 4 out]
              }
              frame False {
              }
            }
          }
          frame "Minimize", "Minimized" {
            w302 = T1."Minimized" ("State")
            n114 = property class="VI"(reference=w308, error in=w307) -> (reference out=w305:refnum<vi>, error out=w306:errorcluster, "FP.State"=w304:T1)
            n115 = Not Equal?(x=w304, y=w302) -> (x != y?=w303:bool)
            n116 = case shown="True" w303 {
              tunnel: [w313 w314] -> w309
              tunnel: w306 -> [w312 w314]
              tunnel: w305 -> [w311 _]
              tunnel: w302 -> [w310 _]
              frame True {
                n117 = invoke class="VI" method="FP.Open"(reference=w311, error in=w312, "State"=w310) -> (error out=w313:errorcluster)  [unwired: 2 in, 4 out]
              }
              frame False {
              }
            }
          }
          frame "Maximize", "Maximized" {
            w315 = T1."Maximized" ("State")
            n118 = property class="VI"(reference=w321, error in=w320) -> (reference out=w318:refnum<vi>, error out=w319:errorcluster, "FP.State"=w317:T1)
            n119 = Not Equal?(x=w317, y=w315) -> (x != y?=w316:bool)
            n120 = case shown="True" w316 {
              tunnel: [w326 w327] -> w322
              tunnel: w319 -> [w325 w327]
              tunnel: w318 -> [w324 _]
              tunnel: w315 -> [w323 _]
              frame True {
                n121 = invoke class="VI" method="FP.Open"(reference=w324, error in=w325, "State"=w323) -> (error out=w326:errorcluster)  [unwired: 2 in, 4 out]
              }
              frame False {
              }
            }
          }
        }
        n122 = call <vilib>:"Add State(s) to Queue__JKI_lib_State_Machine.vi"("State(s) in (\"\")"=w262) -> ("States Out"=w261:string)  [unwired: 14 in]
      }
      frame "UI: Autoset Arguments" {
        n123 = call "CSM - Revert Arguments-Safe String.vi"("Safe Argurment String"=w339) -> ("Origin Argurment String"=w337:string)  [unwired: 8 in]
        n124 = control-ref of="CSM"() -> (w333:refnum<vi>)
        n125 = call "Remove Comments from Single-line.vi"("single-line text"=w337) -> ("single-line text without comments"=w338:string)  [unwired: 2 in]
        n126 = call "Split Single-line Message.vi"("single-line text"=w338) -> ("state"=w335:string, "args"=w334:string, "source/target"=w330:string)  [unwired: 6 in, 1 out]
        n127 = property on="Property Node" class="CmbBox"(reference=w333) -> (reference out=w331:refnum<vi>, "Strings[]"=w332:string[])  [unwired: 1 in, 1 out]
        n128 = Search 1D Array(1D array=w332, element=w330) -> (index of element=w329:i32)  [unwired: 1 in]
        n129 = Greater Or Equal To 0?(x=w329) -> (x >= 0?=w328:bool)
        n130 = case shown="False" w328 {
          tunnel: w331 -> [_ w344]
          tunnel: w330 -> [_ w343]
          frame False {
          }
          frame True {
            n131 = property on="Property Node" class="CmbBox"(reference=w344, "Value"=w343) -> ()  [unwired: 1 in, 2 out]
          }
        }
        n132 = local write "Arguments"(w334) -> ()
        n133 = local write "CSM 2"(w335) -> ()
      }
      frame "UI: Refresh History List" {
        n134 = Unbundle By Name(w350) -> ("MessageList"=w346:string[])
        n135 = property on="History" class="LstBox (strict)"() -> ("Item Names"=w348:string[], "Value"=w349:i32)  [unwired: 2 in, 2 out]
        n136 = Index Array(array=w348, index=w349) -> (element=w347:string)
        n137 = Search 1D Array(1D array=w346, element=w347) -> (index of element=w345:i32)  [unwired: 1 in]
        n138 = property on="History" class="LstBox (strict)"("Item Names"=w346, "Value"=w345) -> ()  [unwired: 2 in, 2 out]
      }
      frame "UI: Refresh CSM List" {
        n139 = control-ref of="CSM"() -> (w362:refnum<vi>)
        n140 = property on="Property Node" class="CmbBox"(reference=w362) -> (reference out=w354:refnum<vi>, "Value"=w358:string)  [unwired: 1 in, 1 out]
        n141 = call "CSM - List Modules.vi"() -> ("error out"=w361:errorcluster, "Module Names"=w356:string[])  [unwired: 10 in]
        n142 = Search 1D Array(1D array=w356, element=w358) -> (index of element=w360:i32)  [unwired: 1 in]
        n143 = Greater Or Equal To 0?(x=w360) -> (x >= 0?=w359:bool)
        n144 = Index Array(array=w356) -> (element=w357:string)  [unwired: 1 in]
        n145 = Select(t=w358, s=w359, f=w357) -> (s? t:f=w355:string)
        n146 = property on="Property Node" class="CmbBox"(reference=w354, "Strings[]"=w356, "Value"=w355) -> ()  [unwired: 1 in, 2 out]
        n147 = call <vilib>:"Simple Error Handler.vi"("error in (no error)"=w361) -> ()  [unwired: 4 in, 5 out]
      }
      frame "UI: Refresh UI" {
      }
      frame "---------- Macro ----------" {
        # "Do not put any code in this frame.\n(It is a separator no-op. You can make a copy of this frame to create a new Macro frame)"
        n148 = call <vilib>:"Add State(s) to Queue__JKI_lib_State_Machine.vi"("State(s) in (\"\")"=w375) -> ("States Out"=w374:string)  [unwired: 14 in]
      }
      frame "Macro: Initialize" {
        # "Initialization Macro\n(This is called once, when the VI starts)"
        n149 = call <vilib>:"Add State(s) to Queue__JKI_lib_State_Machine.vi"("State(s) in Front (\"\")"="Data: Initialize\nData: Initialize References\nInitialize Core Data\nEvents: Register\nUI: Initialize\nData: Load Arguments Config File\nUI: Front Panel State >> Open\nUI: Refresh CSM List\nUI: Refresh History List\nUI: Refresh UI", "State(s) in (\"\")"=w381) -> ("States Out"=w380:string)  [unwired: 13 in]
      }
      frame "Macro: Exit" {
        # "Exit Macro\n(This is called once, when the VI exits)"
        n150 = Unbundle By Name(w389) -> ("Core.Close Panel on Exit?"=w388:bool)
        n151 = Select(t="UI: Front Panel State >> Close", s=w388, f="") -> (s? t:f=w385:string)
        n152 = call <vilib>:"Add State(s) to Queue__JKI_lib_State_Machine.vi"("State(s) in (\"\")"=w385, "State(s) at Back (\"\")"="Data: Save Arguments Config File\nData: Cleanup\nEvents: Unregister\nExit") -> ("States Out"=w383:string)  [unwired: 13 in]
        n153 = call <vilib>:"Add State(s) to Queue__JKI_lib_State_Machine.vi"("State(s) in Front (\"\")"=w383, "State(s) in (\"\")"=w392) -> ("States Out"=w391:string)  [unwired: 13 in]
      }
      frame "---------- Action ----------" {
        # "Template Separator\n(You can make a copy of, or modify, this frame)"
        n154 = call <vilib>:"Add State(s) to Queue__JKI_lib_State_Machine.vi"("State(s) in (\"\")"=w397) -> ("States Out"=w396:string)  [unwired: 14 in]
      }
      frame "Action: Send CSM Message" {
        n155 = local read "CSM"() -> (w400:string)
        n156 = case shown="Default" "CSM 2" {
          selector: "CSM 2" -> [_ w413]
          tunnel: "Arguments" -> [_ w412]
          tunnel: [_ w418] -> w401
          tunnel: w400 -> [_ w411]
          tunnel: [_ w410] -> w399
          tunnel: "RespTMO(ms)" -> [_ w417]
          frame "" {
          }
          frame Default {
            n157 = call "CSM - Send Message and Wait for Reply.vi"("Response Timeout (-2 Using Global Settings)"=w417, "Current Module (\"\" to Generate an ID)"="Tool-Testpnl" ("Current Module(\"\" to generate a ID)"), "Target Module"=w411, "Arguments (\"\")"=w412, "State"=w413) -> ("error out"=w418:errorcluster, "Response"=→"Response":string)  [unwired: 4 in, 1 out]
            n158 = call-poly "Build Message with Arguments++.vi"("State With Arguments"=w413, "Arguments (\"\")"=w412, "Target Module (\"\")"=w411) -> ("CSM Message String"=w415:string)  [unwired: 12 in]
            n159 = call "CSM - Make String Arguments Safe.vi"("Argurment String"=w415) -> ("Safe Argurment String"=w414:string)  [unwired: 8 in]
            n160 = call <vilib>:"Build State String with Arguments__JKI_lib_State_Machine.vi"("Arguments (\"\")"=w414, "State"="Data: Update Message List" ("State(s) in Front (\"\")")) -> ("State with Arguments"=w409:string)  [unwired: 4 in]
            n161 = call <vilib>:"Add State(s) to Queue__jki_lib_state_machine.vi"("State(s) in (\"\")"=w409, "State(s) at Back (\"\")"="UI: Refresh History List\nData: Save Arguments Config File" ("State(s) in Front (\"\")")) -> ("States Out"=w410:string)  [unwired: 13 in]
          }
        }
        n162 = call <vilib>:"Add State(s) to Queue__JKI_lib_State_Machine.vi"("State(s) in (\"\")"=w407, "State(s) at Back (\"\")"=w399) -> ("States Out"=w406:string)  [unwired: 13 in]
      }
      frame "Action: Post CSM Message" {
        # "Your code here.\n(You can make a copy of, or modify, this frame)"
        n163 = local read "Arguments"() -> (w422:string)
        n164 = local read "CSM 2"() -> (w421:string)
        n165 = local read "CSM"() -> (w424:string)
        n166 = case shown="Default" w421 {
          selector: w421 -> [_ w435]
          tunnel: w422 -> [_ w434]
          tunnel: [_ w439] -> w425
          tunnel: w424 -> [_ w433]
          tunnel: [_ w432] -> w423
          frame "" {
          }
          frame Default {
            n167 = call "CSM - Post Message.vi"("Current Module (\"\" to Generate an ID)"="Tool-Testpnl" ("Current Module(\"\" to generate a ID)"), "Target Module"=w433, "Arguments (\"\")"=w434, "State"=w435) -> ("error out"=w439:errorcluster)  [unwired: 7 in]
            n168 = call-poly "Build Message with Arguments++.vi"("State With Arguments"=w435, "Arguments (\"\")"=w434, "Target Module (\"\")"=w433) -> ("CSM Message String"=w437:string)  [unwired: 12 in]
            n169 = call "CSM - Make String Arguments Safe.vi"("Argurment String"=w437) -> ("Safe Argurment String"=w436:string)  [unwired: 8 in]
            n170 = call <vilib>:"Build State String with Arguments__JKI_lib_State_Machine.vi"("Arguments (\"\")"=w436, "State"="Data: Update Message List" ("State(s) in Front (\"\")")) -> ("State with Arguments"=w431:string)  [unwired: 4 in]
            n171 = call <vilib>:"Add State(s) to Queue__JKI_lib_State_Machine.vi"("State(s) in (\"\")"=w431, "State(s) at Back (\"\")"="UI: Refresh History List\nData: Save Arguments Config File" ("State(s) in Front (\"\")")) -> ("States Out"=w432:string)  [unwired: 13 in]
          }
        }
        n172 = call <vilib>:"Add State(s) to Queue__JKI_lib_State_Machine.vi"("State(s) in (\"\")"=w429, "State(s) at Back (\"\")"=w423) -> ("States Out"=w428:string)  [unwired: 13 in]
      }
    }
  }
